vi "浮动通知2.vi"(10 "通知时间(S)":dbl=3.0, 11 "通知内容":string) -> ()   [LabVIEW 2020]
panel:
  in  "背景颜色":u32(colorbox)
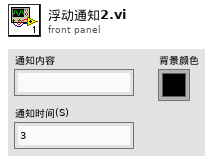
[diagram p1: front panel]
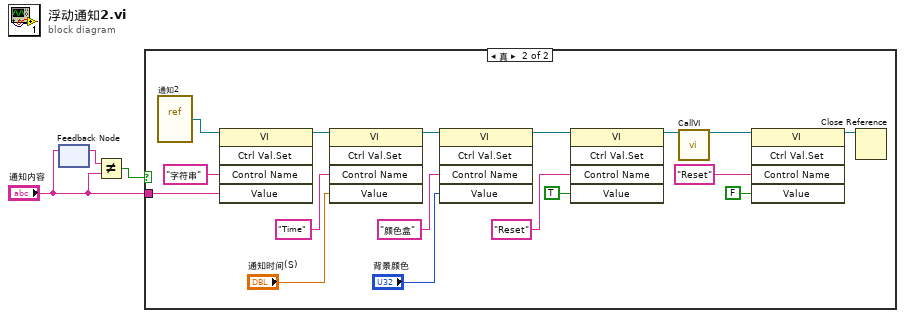
[diagram p0: block diagram]
diagram:
  n1 = feedback-in #1("通知内容") -> ()
  n2 = feedback #1() -> (w2:string)  [unwired: 1 in]
  n3 = Not Equal?(x=w2, y="通知内容") -> (x != y?=w3:bool)
  n4 = case shown="真" w3 {
    tunnel: "通知内容" -> [_ w5]
    frame False {
    }
    frame True {
      n5 = vi-ref "通知2.vi"() -> (w4:refnum<vi>)
      n6 = invoke class="VI" method="Ctrl Val.Set"(reference=w4, "Control Name"="字符串" ("控件名"), "Value"=w5) -> (reference out=w19:refnum<vi>)  [unwired: 2 in, 4 out]
      n7 = invoke class="VI" method="Ctrl Val.Set"(reference=w19, "Control Name"="Time" ("控件名"), "Value"="通知时间(S)") -> (reference out=w9:refnum<vi>)  [unwired: 2 in, 4 out]
      n8 = invoke class="VI" method="Ctrl Val.Set"(reference=w9, "Control Name"="颜色盒" ("控件名"), "Value"="背景颜色") -> (reference out=w8:refnum<vi>)  [unwired: 2 in, 4 out]
      n9 = invoke class="VI" method="Ctrl Val.Set"(reference=w8, "Control Name"="Reset" ("控件名"), "Value"=TRUE) -> (reference out=w11:refnum<vi>)  [unwired: 2 in, 4 out]
      n10 = call "CallVI.vi"("VI引用"=w11) -> ("VI引用输出"=w10:refnum<vi>)  [unwired: 12 in, 2 out]
      n11 = invoke class="VI" method="Ctrl Val.Set"(reference=w10, "Control Name"="Reset" ("控件名"), "Value"=FALSE) -> (reference out=w12:refnum<vi>)  [unwired: 2 in, 4 out]
      n12 = Close Reference(reference=w12) -> ()  [unwired: 1 in, 1 out]
    }
  }
